vi "Stop Core.vi"(10 "final error code":i32, 11 "Mediator in":refnum<class "BusMediator.lvclass">) -> (3 "Mediator out":refnum<class "BusMediator.lvclass">)   [LabVIEW 2017, in "BusMediator.lvclass"]
doc: "(<B>Filename</B>: Actor Framework.lvlib:Actor.lvclass:Stop Core.vi)\n\nDefines what the actor does before it stops. Use the <B>final error code</B> input to determine whether the actor shut down in response to an error.\n\nBy default, this method does nothing. A descendant class may override it to define behavior, such as shutting down any processes the actor initiated in its override of the Actor Core method."
uses:
  BusMediator.lvclass
  <vilib>/Composed/GPM Packages/mva-framework/Source/Framework/IMediator/IMediator/IMediator.lvclass
  <vilib>/ActorFramework/Stop Msg/Stop Msg.lvclass
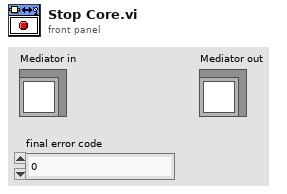
[diagram p1: front panel]
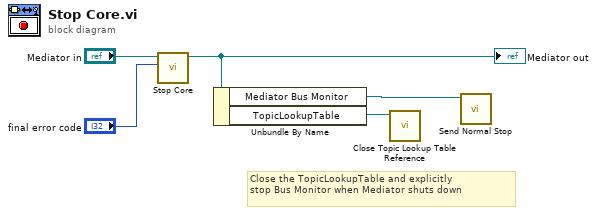
[diagram p0: block diagram]
diagram:
  # "Close the TopicLookupTable and explicitly\nstop Bus Monitor when Mediator shuts down"
  n1 = call-parent "Stop Core.vi"("final error code"="final error code", "Mediator In"="Mediator in") -> ("Mediator Out"=w3:refnum<class "BusMediator.lvclass">)  [unwired: 9 in]
  "Mediator out" <- w3
  n2 = Unbundle By Name(w3) -> ("Mediator Bus Monitor"=w1:refnum<class "Message Enqueuer.lvclass">, "TopicLookupTable"=w2:refnum<data-value>)
  n3 = call "Close Topic Lookup Table Reference.vi"("TopicLookupTable"=w2) -> ()  [unwired: 10 in, 1 out]
  n4 = call <vilib>:"Send Normal Stop.vi"("Message Enqueuer"=w1) -> ()  [unwired: 10 in, 1 out]
